vi "Waveform Results Channels.vi"(8 "error in (no error)":errorcluster, 11 "Node Ptr":T1 format="%.0x") -> (0 "error out":errorcluster)   [LabVIEW 2015, in "Waveform-Processing-Custom-Device System Explorer.lvlib"]
uses:
  Waveform-Processing-Custom-Device System Explorer.lvlib
  <vilib>/NI Veristand/Custom Device API/Custom Device Item Ref.ctl
  <vilib>/NI VeriStand/Custom Device API/Custom Device API.lvlib
panel:
  in  "SHDocVw.IWebBrowser":refnum<k7>(container)
  in  "Specific Header":cluster{"Section Name":string}={"Section Name"="Specific Page Settings"}
  in  "General Header":cluster{"Section Name":string}={"Section Name"="General Page Settings"}
  in  "Description":string
  in  "Name":string
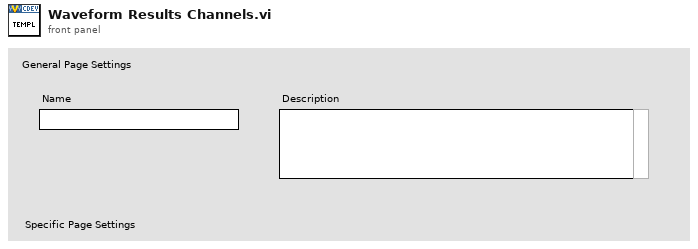
[diagram p1: front panel]
types:
  T1 = typedef "Custom Device API.lvlib/Custom Device Item Ref.ctl" = u64
  T2 = typedef "Custom Device API.lvlib/Custom Device Item Info.ctl" = cluster{"Name":string, "Is Channel":bool, "GUID":string, "Is Waveform":bool}
  T3 = typedef "Custom Device API.lvlib/Custom Device Commands.ctl" = enum16{"Default", "Item renamed", "Shutdown", "Dynamic button pressed"}
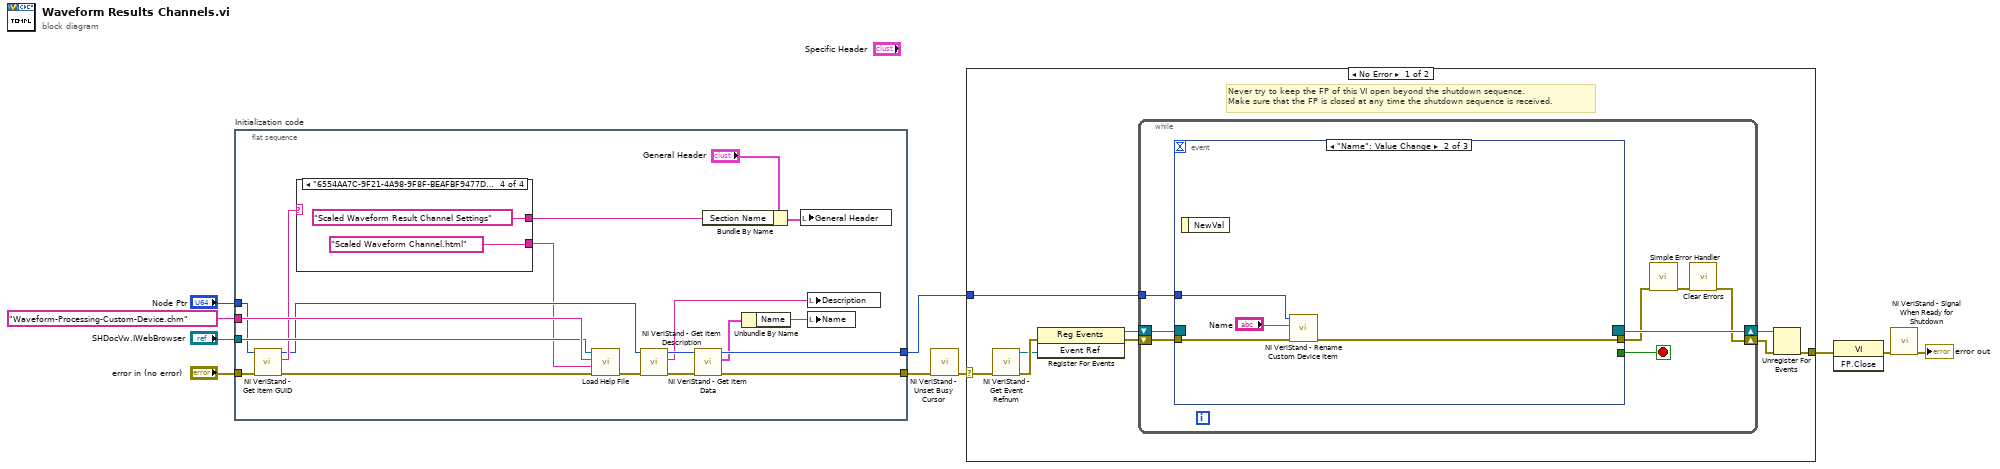
[diagram p0: block diagram]
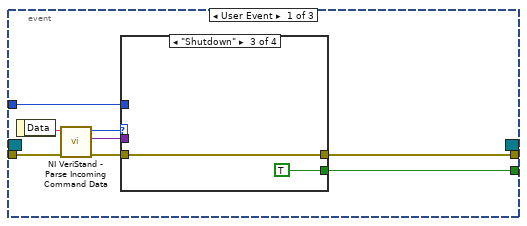
[diagram p2: hidden frame]
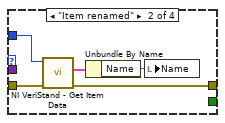
[diagram p4: hidden frame]
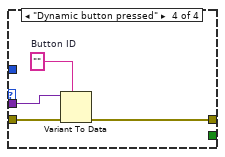
[diagram p5: hidden frame]
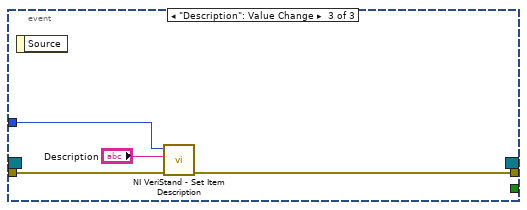
[diagram p6: hidden frame]
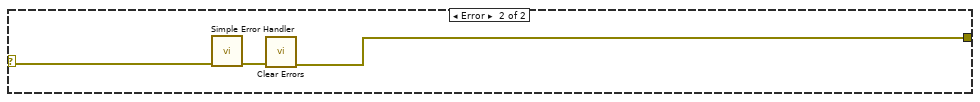
[diagram p7: hidden frame]
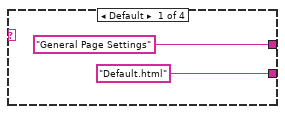
[diagram p8: hidden frame]
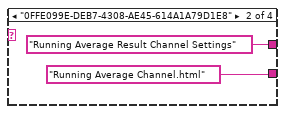
[diagram p9: hidden frame]
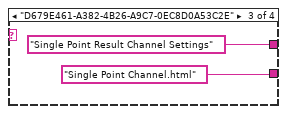
[diagram p10: hidden frame]
diagram:
  n1 = flat-sequence "Initialization code" {
    tunnel: "error in (no error)" -> [w14]
    tunnel: "Node Ptr" -> [w17]
    tunnel: [w25] -> w6
    tunnel: [w29] -> w3
    tunnel: "SHDocVw.IWebBrowser" -> [w23]
    tunnel: "Waveform-Processing-Custom-Device.chm" ("CD_CHM_FileName") -> [w24]
    frame #0 {
      n2 = call <vilib>:"NI VeriStand - Get Item GUID.vi"("error in (no error)"=w14, "Item Ref in"=w17) -> ("error out"=w13:errorcluster, "GUID"=w16:string, "Item Ref out"=w15:T1)  [unwired: 7 in]
      n3 = case shown="\"6554AA7C-9F21-4A98-9F8F-BEAFBF9477D8\"" w16 {
        tunnel: ["General Page Settings" "Running Average Result Channel Settings" "Single Point Result Channel Settings" "Scaled Waveform Result Channel Settings"] -> w18
        tunnel: ["Default.html" ("CD_CHM_Section") "Running Average Channel.html" ("CD_CHM_Section") "Single Point Channel.html" ("CD_CHM_Section") "Scaled Waveform Channel.html" ("CD_CHM_Section")] -> w11
        frame Default {
        }
        frame "0FFE099E-DEB7-4308-AE45-614A1A79D1E8" {
        }
        frame "D679E461-A382-4B26-A9C7-0EC8D0A53C2E" {
        }
        frame "6554AA7C-9F21-4A98-9F8F-BEAFBF9477D8" {
        }
      }
      n4 = call "Load Help File.vi"("error in (no error)"=w13, "HTML File to Load"=w11, "Main CHM File"=w24, "Browser"=w23) -> ("error out"=w12:errorcluster)  [unwired: 7 in]
      n5 = call <vilib>:"NI VeriStand - Get Item Description.vi"("error in (no error)"=w12, "Item Ref in"=w15) -> ("error out"=w27:errorcluster, "Description"=w21:string, "Item Ref out"=w28:T1)  [unwired: 7 out]
      n6 = call <vilib>:"NI VeriStand - Get Item Data.vi"("error in (no error)"=w27, "Item Ref in"=w28) -> ("error out"=w25:errorcluster, "Item Info"=w26:T2, "Item Ref out"=w29:T1)  [unwired: 7 out]
      n7 = Bundle By Name(cluster="General Header", "Section Name"=w18) -> (w19:cluster{"Section Name":string})
      n8 = Unbundle By Name(w26) -> ("Name"=w22:string)
      n9 = local write "General Header"(w19) -> ()
      n10 = local write "Description"(w21) -> ()
      n11 = local write "Name"(w22) -> ()
    }
  }
  n12 = call <vilib>:"NI VeriStand - Unset Busy Cursor.vi"("error in (no error)"=w6) -> ("error out"=w5:errorcluster)  [unwired: 10 out]
  n13 = case shown="No Error" w5 {
    selector: w5 -> [w38 w85]
    tunnel: [w43 w83] -> w10
    tunnel: w3 -> [w39 _]
    frame No Error {
      # "Never try to keep the FP of this VI open beyond the shutdown sequence.\nMake sure that the FP is closed at any time the shutdown sequence is received."
      n14 = call <vilib>:"NI VeriStand - Get Event Refnum.vi"("error in (no error)"=w38) -> ("error out"=w46:errorcluster, "Event Ref"=w42:refnum<user-event>)  [unwired: 9 out]
      n15 = register-events(error in=w46, w42) -> (reference out=w40:refnum<event-registration>, error out=w41:errorcluster)  [unwired: 1 in]
      n16 = while {
        tunnel: w39 -> [w50]
        shift-right: [w47] -> w44
        shift-left: w41 -> [w53]
        shift-right: [w54] -> w45
        shift-left: w40 -> [w52]
        stop <- w51 stop-if-true
        n17 = event shown="[1] \"Name\": Value Change" {
          selector: w52 -> [_ _ _]
          dyn-events: [_ _ _] -> w54
          timeout: _ -> [_ _ _]
          tunnel: w53 -> [w62 w78 w81]
          tunnel: [w58 _ _] -> w51
          tunnel: [w57 w77 w80] -> w49
          tunnel: w50 -> [w56 w76 w82]
          event User Event {
            n18 = event-data() -> ("Data"=w61:string)  [unwired: 1 out]
            n19 = call <vilib>:"NI VeriStand - Parse Incoming Command Data.vi"("error in (no error)"=w62, "Incoming data"=w61) -> ("error out"=w60:errorcluster, "Outgoing data"=w55:variant, "Action"=w59:T3)  [unwired: 7 out]
            n20 = case shown="\"Shutdown\"" w59 {
              tunnel: w60 -> [w63 w68 w69 w74]
              tunnel: [_ _ TRUE _] -> w58
              tunnel: [w63 w65 w69 w71] -> w57
              tunnel: w56 -> [_ w67 _ _]
              tunnel: w55 -> [_ _ _ w73]
              frame "Default", Default {
              }
              frame "Item renamed" {
                n21 = call <vilib>:"NI VeriStand - Get Item Data.vi"("error in (no error)"=w68, "Item Ref in"=w67) -> ("error out"=w65:errorcluster, "Item Info"=w66:T2)  [unwired: 8 out]
                n22 = Unbundle By Name(w66) -> ("Name"=w64:string)
                n23 = local write "Name"(w64) -> ()
              }
              frame "Shutdown" {
              }
              frame "Dynamic button pressed" {
                w72 = ""  # Button ID
                n24 = Variant To Data(error in=w74, type=w72, Variant=w73) -> (error out=w71:errorcluster)  [unwired: 1 out]
              }
            }
          }
          event "Name": Value Change {
            n25 = event-data() -> ()  [unwired: 2 out]
            n26 = call <vilib>:"NI VeriStand - Rename Custom Device Item.vi"("error in (no error)"=w78, "New Name"="Name", "Item Ref in"=w76) -> ("error out"=w77:errorcluster)  [unwired: 1 in, 7 out]
          }
          event "Description": Value Change {
            n27 = event-data() -> ()  [unwired: 2 out]
            n28 = call <vilib>:"NI VeriStand - Set Item Description.vi"("error in (no error)"=w81, "Description"="Description", "Item Ref in"=w82) -> ("error out"=w80:errorcluster)  [unwired: 8 out]
          }
        }
        n29 = call <vilib>:"Simple Error Handler.vi"("error in (no error)"=w49) -> ("error out"=w48:errorcluster)  [unwired: 1 in, 7 out]
        n30 = call <vilib>:"Clear Errors.vi"("error in (no error)"=w48) -> ("error out"=w47:errorcluster)  [unwired: 1 in, 5 out]
      }
      n31 = Unregister For Events(event registration refnum=w45, error in=w44) -> (error out=w43:errorcluster)
    }
    frame Error {
      n32 = call <vilib>:"Simple Error Handler.vi"("error in (no error)"=w85) -> ("error out"=w84:errorcluster)  [unwired: 1 in, 7 out]
      n33 = call <vilib>:"Clear Errors.vi"("error in (no error)"=w84) -> ("error out"=w83:errorcluster)  [unwired: 1 in, 5 out]
    }
  }
  n34 = invoke class="VI" method="FP.Close"(error in=w10) -> (error out=w9:errorcluster)  [unwired: 2 in, 2 out]
  n35 = call <vilib>:"NI VeriStand - Signal When Ready for Shutdown.vi"("error in (no error)"=w9) -> ("error out"=→"error out":errorcluster)  [unwired: 10 out]
